vi "ex_2.vi"() -> ()   [LabVIEW 2020]
panel:
  out "Boolean":bool
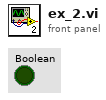
[diagram p1: front panel]
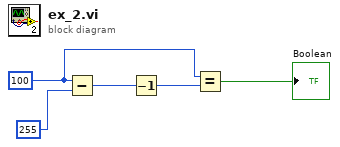
[diagram p0: block diagram]
diagram:
  w2 = u8 100
  n1 = Subtract(x=w2, y=u8 255) -> (x-y=w4:u8)
  n2 = Decrement(x=w4) -> (x-1=w3:u8)
  n3 = Equal?(x=w2, y=w3) -> (x = y?=→"Boolean":bool)
